vi "Send Release Aquirer.vi"(8 "error in (no error)":errorcluster, 10 "Aquirer Index":i32, 11 "Message Enqueuer":refnum<class "Message Enqueuer.lvclass">) -> (0 "error out":errorcluster)   [LabVIEW 2020, in "Instrument Handler.lvlib" / "Release Aquirer Msg.lvclass"]
doc: "This VI sends the message to an actor on High priority."
uses:
  Release Aquirer Msg.lvclass
  PPL/HDH.Actor Framework.Core.Actor.lvlibp/1abvi3w/vi.lib/ActorFramework/Message Enqueuer/Message Enqueuer.lvclass
  PPL/HDH.Actor Framework.Core.Actor.lvlibp/1abvi3w/vi.lib/ActorFramework/Message Enqueuer/Message Priority.ctl
  Release Aquirer Msg.lvclass/Release Aquirer Msg.ctl
  C:/Current projects/WS/PPL/HDH.Actor Framework.Core.Actor.lvlibp/1abvi3w/vi.lib/ActorFramework/Message/Message.lvclass
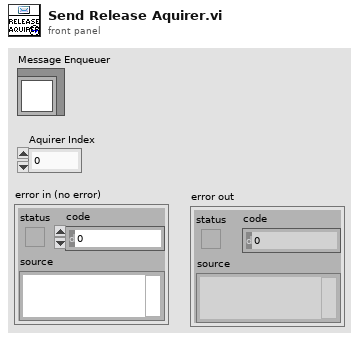
[diagram p1: front panel]
types:
  T1 = typedef "HDH.Actor Framework.Core.Actor.lvlibp/Message Enqueuer.lvclass/Message Priority.ctl" = enum16{"Low", "Normal", "High"}
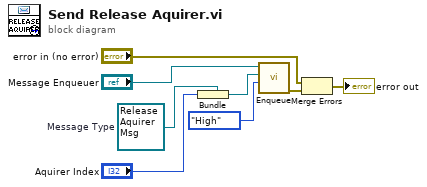
[diagram p0: block diagram]
diagram:
  w6 = refnum<class "Release Aquirer Msg.lvclass"> refnum  # Message Type
  n1 = Bundle(cluster=w6, "Aquirer Index") -> (w5:refnum<class "Release Aquirer Msg.lvclass">)
  n2 = call "Enqueue.vi"("Message Priority (Normal)"=Message_Priority."High", "Message"=w5, "Message Enqueuer in"="Message Enqueuer") -> ("error out"=w7:errorcluster)  [unwired: 7 in, 1 out]
  n3 = Merge Errors("error in (no error)", w7) -> (→"error out":errorcluster)
